vi "Stop.vi"(8 "error in (no error)":errorcluster, 11 "FitterBase in":refnum<class "CorrFactor.lvclass">) -> (0 "error out":errorcluster, 3 "FitterBase out":refnum<class "CorrFactor.lvclass">)   [LabVIEW 2018, in "AnalysisPlugins.lvlib" / "CorrFactor.lvclass"]
uses:
  CorrFactor.lvclass
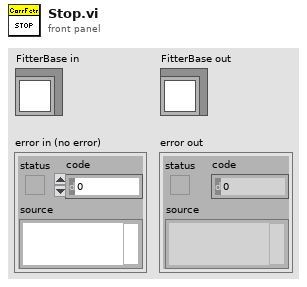
[diagram p1: front panel]
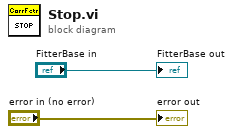
[diagram p0: block diagram]
diagram:
  "error out" <- "error in (no error)"
  "FitterBase out" <- "FitterBase in"
